vi "readInageData.vi"(8 "error in (no error)":errorcluster, 11 "file (use dialog)":path) -> (0 "error out":errorcluster, 1 "format":i32, 3 "Bytes":u8[](array[numeric]))   [LabVIEW 2017, in "LabVIEW NPOI.lvlib" / "MS-Excel.lvclass"]
uses:
  MS-Excel.lvclass
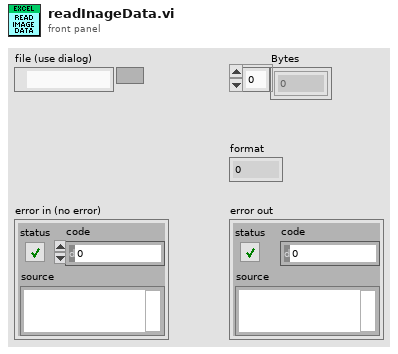
[diagram p1: front panel]
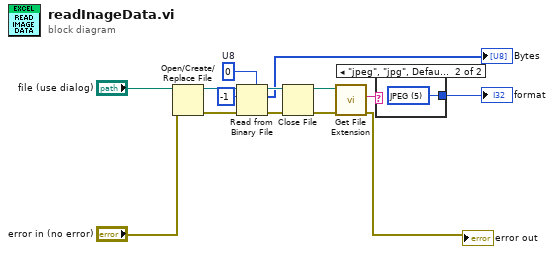
[diagram p0: block diagram]
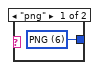
[diagram p2: hidden frame]
diagram:
  w4 = u8 0  # U8
  n1 = Open/Create/Replace File(file path (use dialog)="file (use dialog)", error in="error in (no error)") -> (refnum out=w2:refnum<file>, error out=w1:errorcluster)  [unwired: 4 in, 1 out]
  n2 = Read from Binary File(5:w4, 8:w1, 10:-1 ("count (1)"), 11:w2) -> (0:w6:errorcluster, 2:→"Bytes":u8[], 3:w7:refnum<file>)  [unwired: 2 in, 1 out]
  n3 = Close File(refnum=w7, error in=w6) -> (path=w9:path, error out=w10:errorcluster)
  n4 = call <vilib>:"Get File Extension.vi"("error in (no error)"=w10, "file"=w9) -> ("error out"=→"error out":errorcluster, "lowercase file extension"=w11:string)  [unwired: 5 in, 3 out]
  n5 = case shown="\"jpeg\", \"jpg\", Default" w11 {
    tunnel: [w15 w16] -> w12
    frame "png" {
      w15 = 6 items=["None"=0, "EMF"=2, "WMF"=3, "PICT"=4, "JPEG"=5, "PNG"=6, "DIB"=7] ("format")
    }
    frame "jpeg", "jpg", Default {
      w16 = 5 items=["None"=0, "EMF"=2, "WMF"=3, "PICT"=4, "JPEG"=5, "PNG"=6, "DIB"=7] ("format")
    }
  }
  "format" <- w12
